vi "ReadWrite LoopStats.vi"(5 "Late":bool, 6 "Iteration Duration":i64, 7 "Mode":T1, 8 "error in (no error)":errorcluster, 11 "RT Data in":T2 {"Label Transfer Config"."Block Data Refs"."Data Reference" format="%.0x"; "Status Config"."HWOut Dur Ref" format="%.0x"; "Status Config"."HWIn Dur Ref" format="%.0x"; "Status Config"."HWOut Count Ref" format="%.0x"; "Status Config"."HWIn Count Ref" format="%.0x"; "Status Config"."Error Data Ref" format="%.0x"; "HWOutput Channels"."Labels Settings"."Driver Data"."Num Bits" min=1 max=32; "HWOutput Channels"."Labels Settings"."Driver Data"."Start Bit" min=8 max=31; "HWOutput Channels"."Labels Settings"."Block Data Refs"."Data Reference" format="%.0x"; "HWOutput Channels"."Labels Settings"."Label" format="%.0o"; "HWInput Channels"."Labels Settings"."Driver Data"."Num Bits" min=1 max=32; "HWInput Channels"."Labels Settings"."Driver Data"."Start Bit" min=8 max=31; "HWInput Channels"."Labels Settings"."Block Data Refs"."Data Reference" format="%.0x"; "HWInput Channels"."Labels Settings"."Label" format="%.0o"}) -> (0 "error out":errorcluster, 3 "RT Data out":T2 {"Label Transfer Config"."Block Data Refs"."Data Reference" format="%.0x"; "Status Config"."HWOut Dur Ref" format="%.0x"; "Status Config"."HWIn Dur Ref" format="%.0x"; "Status Config"."HWOut Count Ref" format="%.0x"; "Status Config"."HWIn Count Ref" format="%.0x"; "Status Config"."Error Data Ref" format="%.0x"; "HWOutput Channels"."Labels Settings"."Driver Data"."Num Bits" min=1 max=32; "HWOutput Channels"."Labels Settings"."Driver Data"."Start Bit" min=8 max=31; "HWOutput Channels"."Labels Settings"."Block Data Refs"."Data Reference" format="%.0x"; "HWOutput Channels"."Labels Settings"."Label" format="%.0o"; "HWInput Channels"."Labels Settings"."Driver Data"."Num Bits" min=1 max=32; "HWInput Channels"."Labels Settings"."Driver Data"."Start Bit" min=8 max=31; "HWInput Channels"."Labels Settings"."Block Data Refs"."Data Reference" format="%.0x"; "HWInput Channels"."Labels Settings"."Label" format="%.0o"})   [LabVIEW 2011, in "AIT 1553 Custom Device.lvlib"]
uses:
  AIT 1553 Custom Device.lvlib
  RT Controls/RT Data.ctl
  RT Controls/RT HW Channel.ctl
  RT Controls/RT Label Settings.ctl
  Controls and Global/Label.ctl
  Controls and Global/transferPeriod.ctl
  <vilib>/NI Veristand/Custom Device API/Block Data Reference.ctl
  <vilib>/NI Veristand/Custom Device API/Data Reference.ctl
  RT Controls/Driver Data.ctl
  Controls and Global/Start Bit.ctl
  Controls and Global/Number of Bits.ctl
  RT Controls/Error Qs.ctl
  RT Controls/Status Channels Config.ctl
  RT Controls/FIFO.ctl
  RT Controls/Label Transfer Config.ctl
  <userlib>/ARINC-429/vi/enum/Owl429HardwareSource.ctl
  RT Controls/ReadWrite Selector.ctl
  <vilib>/NI Veristand/Custom Device API/Global Data Refs.vi
  <vilib>/NI Veristand/Custom Device API/Custom Device API.lvlib
  <userlib>/ARINC-429/Owl429.lvlib
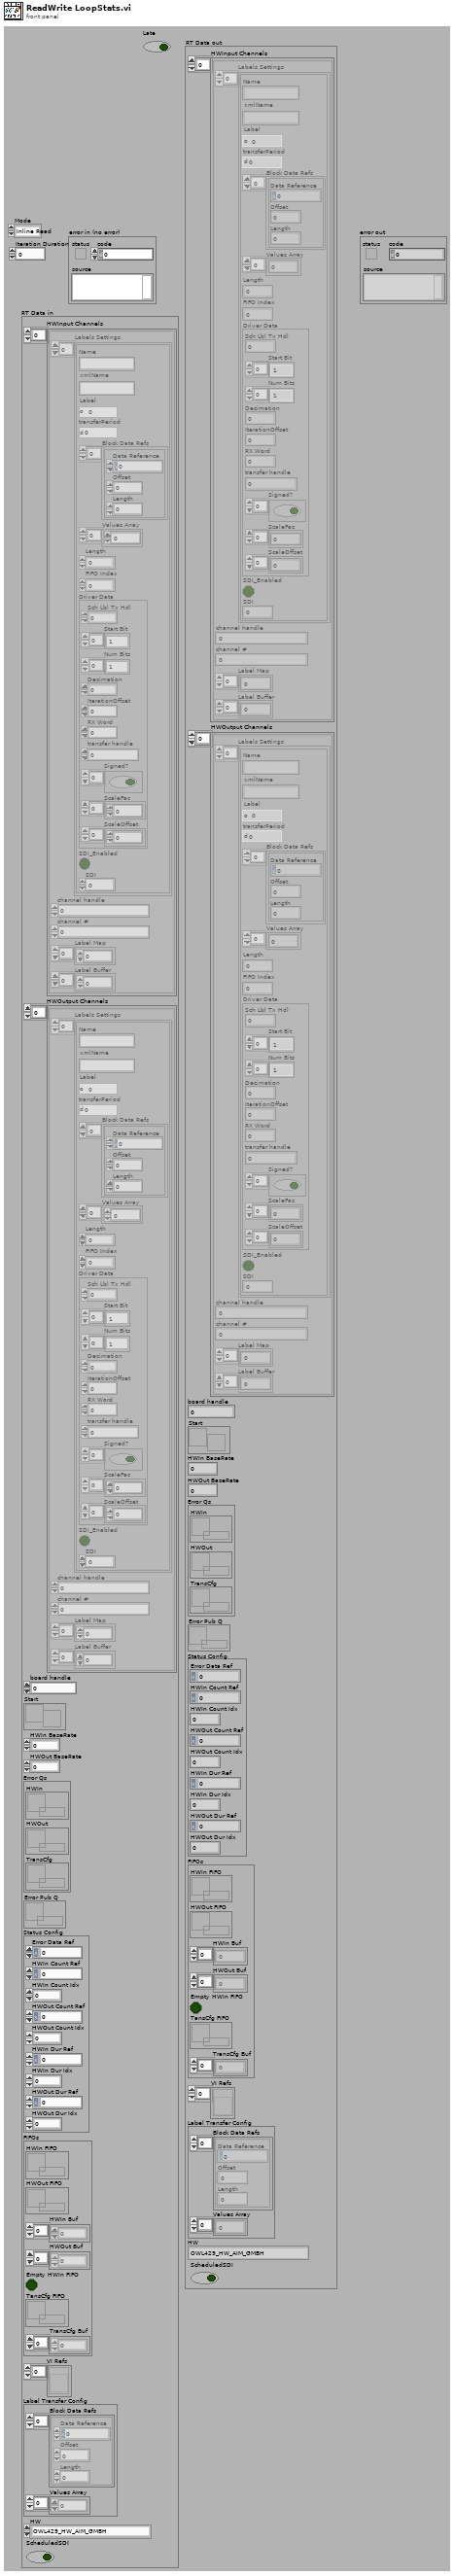
[diagram p1: front panel]
types:
  T1 = typedef "AIT 1553 Custom Device.lvlib/ReadWrite Selector.ctl" = enum16{"Inline Read", "Inline Write", "Async HWIn", "Async HWOut"}
  T2 = typedef "AIT 1553 Custom Device.lvlib/RT Data.ctl" = cluster{"HWInput Channels":T3[], "HWOutput Channels":T3[], "board handle":u32, "Start":refnum<notifier>, "HWIn BaseRate":i64, "HWOut BaseRate":i64, "Error Qs":T12, "Error Pub Q":refnum<queue>, "Status Config":T13, "FIFOs":T14, "VI Refs":refnum<vi>[], "Label Transfer Config":T15, "HW":T16, "ScheduledSDI":bool}
  T3 = typedef "AIT 1553 Custom Device.lvlib/RT HW Channel.ctl" = cluster{"Labels Settings":T4[], "channel handle":u32, "channel #":u16, "Label Map":i32[], "Label Buffer":u32[]}
  T4 = typedef "AIT 1553 Custom Device.lvlib/RT Label Settings.ctl" = cluster{"Name":string, "xmlName":string, "Label":T5, "transferPeriod":T6, "Block Data Refs":T7[], "Values Array":dbl[], "Length":i32, "FIFO Index":i32, "Driver Data":T9, "SDI_Enabled":bool, "SDI":u8}
  T5 = typedef "AIT 1553 Custom Device.lvlib/Label.ctl" = u8
  T6 = typedef "AIT 1553 Custom Device.lvlib/transferPeriod.ctl" = u32
  T7 = typedef "Custom Device API.lvlib/Block Data Reference.ctl" = cluster{"Data Reference":T8, "Offset":i32, "Length":i32}
  T8 = typedef "Custom Device API.lvlib/Data Reference.ctl" = i32
  T9 = typedef "AIT 1553 Custom Device.lvlib/Driver Data.ctl" = cluster{"Sch Lbl Tx Hdl":u32, "Start Bit":T10[], "Num Bits":T11[], "Decimation":i32, "IterationOffset":i32, "RX Word":u32, "transfer handle":u32, "Signed?":bool[], "ScaleFac":dbl[], "ScaleOffset":dbl[]}
  T10 = typedef "AIT 1553 Custom Device.lvlib/Start Bit.ctl" = i32
  T11 = typedef "AIT 1553 Custom Device.lvlib/Number of Bits.ctl" = i32
  T12 = typedef "AIT 1553 Custom Device.lvlib/Error Qs.ctl" = cluster{"HWIn":refnum<queue>, "HWOut":refnum<queue>, "TransCfg":refnum<queue>}
  T13 = typedef "AIT 1553 Custom Device.lvlib/Status Channels Config.ctl" = cluster{"Error Data Ref":T8, "HWIn Count Ref":T8, "HWIn Count Idx":i32, "HWOut Count Ref":T8, "HWOut Count Idx":i32, "HWIn Dur Ref":T8, "HWIn Dur Idx":i32, "HWOut Dur Ref":T8, "HWOut Dur Idx":i32}
  T14 = typedef "AIT 1553 Custom Device.lvlib/FIFO.ctl" = cluster{"HWIn FIFO":refnum<k33>, "HWOut FIFO":refnum<k33>, "HWIn Buf":dbl[], "HWOut Buf":dbl[], "Empty HWIn FIFO":bool, "TansCfg FIFO":refnum<k33>, "TransCfg Buf":dbl[]}
  T15 = typedef "AIT 1553 Custom Device.lvlib/Label Transfer Config.ctl" = cluster{"Block Data Refs":T7[], "Values Array":dbl[]}
  T16 = typedef "Owl429.lvlib/Owl429HardwareSource.ctl" = enum16{"OWL429_HW_AIM_GMBH", "OWL429_HW_AIT"}
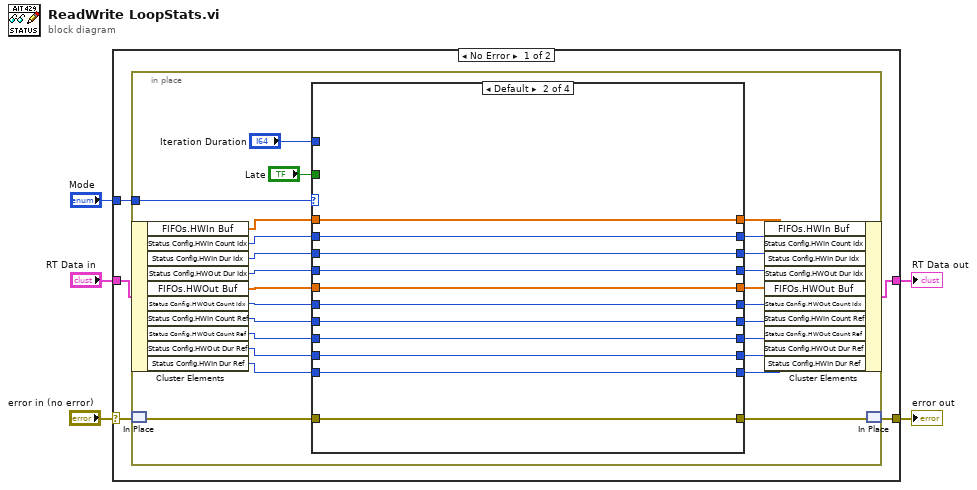
[diagram p0: block diagram]
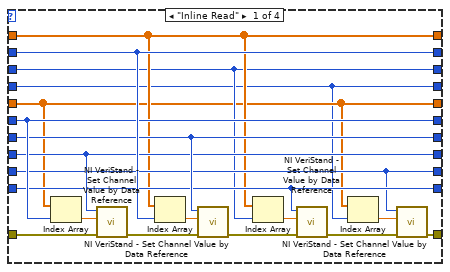
[diagram p2: hidden frame]
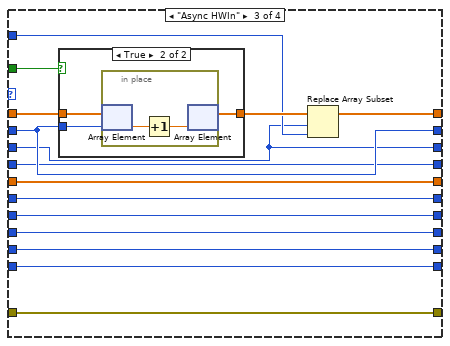
[diagram p3: hidden frame]
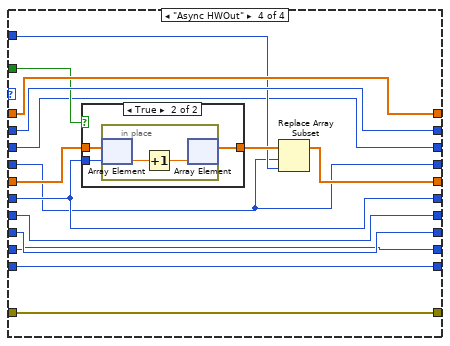
[diagram p5: hidden frame]
diagram:
  n1 = case shown="No Error" "error in (no error)" {
    selector: "error in (no error)" -> [w9 w109]
    tunnel: "RT Data in" -> [w10 w108]
    tunnel: [w8 w108] -> w3
    tunnel: [w7 w109] -> w2
    tunnel: "Mode" -> [w6 _]
    frame No Error {
      n2 = in-place {
        in-place-border: w6 -> [w27]
        n3 = in-place-cluster #1(w10) -> ("FIFOs.HWIn Buf"=w35:dbl[], "Status Config.HWIn Count Idx"=w34:i32, "Status Config.HWIn Dur Idx"=w19:i32, "Status Config.HWOut Dur Idx"=w15:i32, "FIFOs.HWOut Buf"=w33:dbl[], "Status Config.HWOut Count Idx"=w32:i32, "Status Config.HWIn Count Ref"=w29:T8, "Status Config.HWOut Count Ref"=w28:T8, "Status Config.HWOut Dur Ref"=w13:T8, "Status Config.HWIn Dur Ref"=w11:T8)
        n4 = in-place-match #2(w9) -> (w31:errorcluster)
        n5 = case shown="Default" w27 {
          tunnel: w35 -> [w41 w59 w74 w98]
          tunnel: w34 -> [w50 w60 w73 w97]
          tunnel: w33 -> [w37 w61 w80 w95]
          tunnel: w32 -> [w49 w62 w79 w94]
          tunnel: w31 -> [w54 w65 w76 w99]
          tunnel: [w45 w65 w76 w99] -> w30
          tunnel: w29 -> [w48 w63 w77 w100]
          tunnel: w28 -> [w47 w64 w78 w101]
          tunnel: [w47 w64 w78 w101] -> w26
          tunnel: [w48 w63 w77 w100] -> w25
          tunnel: [w49 w62 w79 w94] -> w24
          tunnel: [w37 w61 w80 w92] -> w23
          tunnel: [w50 w60 w73 w97] -> w22
          tunnel: [w41 w59 w71 w98] -> w21
          tunnel: "Late" -> [_ _ w75 w96]
          tunnel: w19 -> [w39 w57 w69 w90]
          tunnel: "Iteration Duration" -> [_ _ w70 w91]
          tunnel: [w39 w57 w69 w90] -> w17
          tunnel: [w36 w58 w68 w89] -> w16
          tunnel: w15 -> [w36 w58 w68 w89]
          tunnel: [w42 w56 w67 w88] -> w14
          tunnel: w13 -> [w42 w56 w67 w88]
          tunnel: [w43 w55 w66 w87] -> w12
          tunnel: w11 -> [w43 w55 w66 w87]
          frame "Inline Read" {
            n6 = Index Array(array=w37, index=w49) -> (element=w52:dbl)
            n7 = call <vilib>:"NI VeriStand - Set Channel Value by Data Reference.vi"("error in (no error)"=w54, "Value"=w52, "Data Reference in"=w47) -> ("error out"=w51:errorcluster)  [unwired: 8 in]
            n8 = Index Array(array=w41, index=w50) -> (element=w53:dbl)
            n9 = call <vilib>:"NI VeriStand - Set Channel Value by Data Reference.vi"("error in (no error)"=w51, "Value"=w53, "Data Reference in"=w48) -> ("error out"=w46:errorcluster)  [unwired: 8 in]
            n10 = Index Array(array=w41, index=w39) -> (element=w40:dbl)
            n11 = call <vilib>:"NI VeriStand - Set Channel Value by Data Reference.vi"("error in (no error)"=w46, "Value"=w40, "Data Reference in"=w43) -> ("error out"=w44:errorcluster)  [unwired: 8 in]
            n12 = Index Array(array=w37, index=w36) -> (element=w38:dbl)
            n13 = call <vilib>:"NI VeriStand - Set Channel Value by Data Reference.vi"("error in (no error)"=w44, "Value"=w38, "Data Reference in"=w42) -> ("error out"=w45:errorcluster)  [unwired: 8 in]
          }
          frame Default {
          }
          frame "Async HWIn" {
            n14 = case shown="True" w75 {
              tunnel: w74 -> [w81 w84]
              tunnel: w73 -> [_ w83]
              tunnel: [w81 w82] -> w72
              frame False {
              }
              frame True {
                n15 = in-place {
                  n16 = in-place-array #3(w84, w83) -> (w86:dbl)
                  n17 = Increment(x=w86) -> (x+1=w85:dbl)
                  n18 = in-place-array #3(w85) -> (w82:dbl[])  [unwired: 1 out]
                }
              }
            }
            n19 = Replace Array Subset(array=w72, new element=w70, index=w69) -> (w71:dbl[])
          }
          frame "Async HWOut" {
            n20 = case shown="True" w96 {
              tunnel: [w102 w105] -> w93
              tunnel: w95 -> [w102 w104]
              tunnel: w94 -> [_ w103]
              frame False {
              }
              frame True {
                n21 = in-place {
                  n22 = in-place-array #4(w104, w103) -> (w107:dbl)
                  n23 = Increment(x=w107) -> (x+1=w106:dbl)
                  n24 = in-place-array #4(w106) -> (w105:dbl[])  [unwired: 1 out]
                }
              }
            }
            n25 = Replace Array Subset(array=w93, new element=w91, index=w89) -> (w92:dbl[])
          }
        }
        n26 = in-place-cluster #1("FIFOs.HWIn Buf"=w21, "Status Config.HWIn Count Idx"=w22, "Status Config.HWIn Dur Idx"=w17, "Status Config.HWOut Dur Idx"=w16, "FIFOs.HWOut Buf"=w23, "Status Config.HWOut Count Idx"=w24, "Status Config.HWIn Count Ref"=w25, "Status Config.HWOut Count Ref"=w26, "Status Config.HWOut Dur Ref"=w14, "Status Config.HWIn Dur Ref"=w12) -> (w8:T2)
        n27 = in-place-match #2(w30) -> (w7:errorcluster)
      }
    }
    frame Error {
    }
  }
  "error out" <- w2
  "RT Data out" <- w3
